vi "Unflatten.vi"(8 "error in (no error)":errorcluster, 11 "Varian Continuous in":refnum<class "Varian Continuous.lvclass">) -> (0 "error out":errorcluster, 3 "Varian Continuous out":refnum<class "Varian Continuous.lvclass">)   [LabVIEW 2009, in "Varian Continuous.lvclass"]
uses:
  Varian Continuous.lvclass
  Scanner/Scanner.lvclass
  Global/File Locations.vi
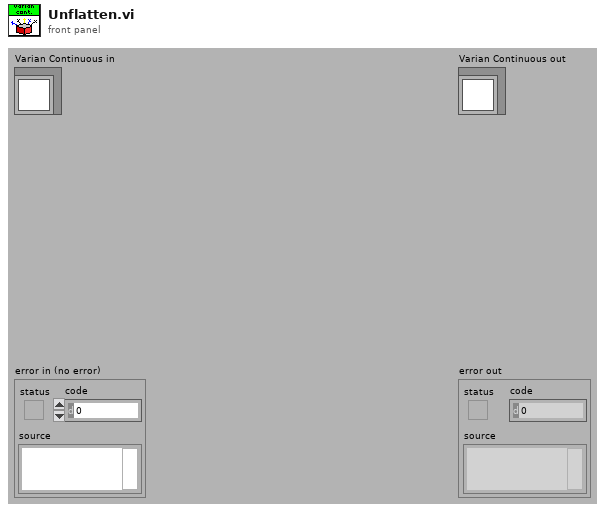
[diagram p1: front panel]
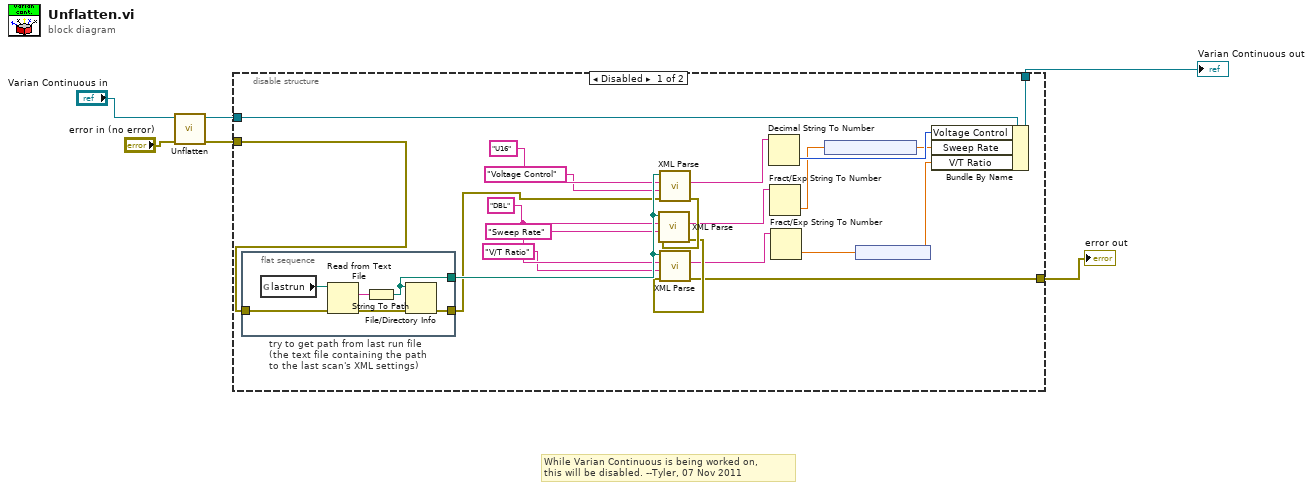
[diagram p0: block diagram]
diagram:
  # "While Varian Continuous is being worked on, \nthis will be disabled. --Tyler, 07 Nov 2011"
  n1 = call-parent "Unflatten.vi"("error in (no error)"="error in (no error)", "Scanner in"="Varian Continuous in") -> ("error out"=w2:errorcluster, "Scanner out"=w6:refnum<class "Varian Continuous.lvclass">)  [unwired: 8 in]
  n2 = disable-structure shown="Disabled" {
    disable-tunnel: w6 -> [w27 w35]
    disable-tunnel: [w26 w35] -> w3
    disable-tunnel: w2 -> [w25 w34]
    disable-tunnel: [w16 w34] -> w1
    frame #0 {
      w22 = "DBL"
      n3 = flat-sequence "try to get path from last run file\n(the text file containing the path\nto the last scan's XML settings)" {
        tunnel: [w33] -> w24
        tunnel: [w29] -> w19
        tunnel: w25 -> [w28]
        frame #0 {
          n4 = global read "File Locations.vi" "lastrun"() -> (w31:path)
          n5 = Read from Text File(file (use dialog)=w31, error in=w28) -> (text=w32:string, error out=w30:errorcluster)  [unwired: 4 out]
          n6 = String To Path(string=w32) -> (path=w33:path)
          n7 = File/Directory Info(path=w33, error in=w30) -> (error out=w29:errorcluster)  [unwired: 6 out]
        }
      }
      n8 = call "XML Parse.vi"("error in (no error)"=w19, "Name String"="Voltage Control", "Type String"="U16", "Path"=w24) -> ("error out"=w18:errorcluster, "String Out"=w13:string)  [unwired: 6 in]
      n9 = call "XML Parse.vi"("error in (no error)"=w18, "Name String"="Sweep Rate", "Type String"=w22, "Path"=w24) -> ("error out"=w17:errorcluster, "String Out"=w12:string)  [unwired: 6 in]
      n10 = call "XML Parse.vi"("error in (no error)"=w17, "Name String"="V/T Ratio", "Type String"=w22, "Path"=w24) -> ("error out"=w16:errorcluster, "String Out"=w11:string)  [unwired: 6 in]
      n11 = Decimal String To Number(string=w13) -> (number=w14:i32)  [unwired: 2 in, 1 out]
      n12 = Fract/Exp String To Number(string=w12) -> (number=w10:dbl)  [unwired: 3 in, 1 out]
      n13 = Fract/Exp String To Number(string=w11) -> (number=w9:dbl)  [unwired: 3 in, 1 out]
      n14 = node(w10) -> (w8:dbl[unit])
      n15 = node(w9) -> (w7:dbl[unit])
      n16 = Bundle By Name(cluster=w27, "Voltage Control"=w14, "Sweep Rate"=w8, "V/T Ratio"=w7) -> (w26:refnum<class "Varian Continuous.lvclass">)
    }
    frame #1 {
    }
  }
  "error out" <- w1
  "Varian Continuous out" <- w3
